vi "Query discriminator level.vi"(8 "error in (no error)":errorcluster, 10 "i (0)":T1, 11 "VISA resource name":refnum<visa-resource-name>) -> (0 "error out":errorcluster, 2 "output":dbl, 3 "VISA resource name out":refnum<visa-resource-name>)   [LabVIEW 2009, in "SR400.lvlib"]
doc: "DL i { ,v }\nThe DL command sets and reads the discriminator\nlevels. i = 0,1, or 2 designates discriminator A,B,\nor T and is required. If v is included, the selected\ndiscriminator level is set to v Volts where -0.3000\n<= V <= 0.3000. The resolution is 0.0002 V (0.2\nmV). If v is absent, the selected discriminator level\nis returned. If the discriminator mode is SCAN,\nthe DL command sets and reads the starting value\nof the level. Changing the level during a scan will\ncause the level to be set to the new value on the\nnext count period. Note that the scan is not reset.\nReading the level during a scan always returns the\nstarting value, not the current value."
uses:
  SR400.lvlib
  Typedefs.llb/Counter.ctl
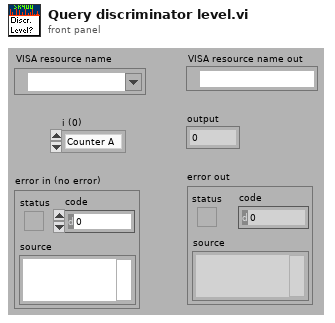
[diagram p1: front panel]
types:
  T1 = typedef "SR400.lvlib/Counter.ctl" = enum16{"Counter A", "Counter B", "Counter T"}
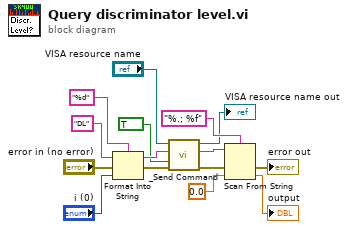
[diagram p0: block diagram]
diagram:
  n1 = Format Into String(format string="%d", initial string="DL" ("command"), error in="error in (no error)", "i (0)") -> (resulting string=w6:string, error out=w5:errorcluster)
  n2 = call "_Send Command.vi"("error in (no error)"=w5, "Query? (F)"=TRUE, "Command"=w6, "VISA resource name"="VISA resource name") -> ("error out"=w2:errorcluster, "Response"=w3:string, "VISA resource name out"=→"VISA resource name out":refnum<visa-resource-name>)  [unwired: 5 out]
  n3 = Scan From String(format string="%.; %f", input string=w3, error in=w2, default 1=0.0 ("default value 1")) -> (error out=→"error out":errorcluster, output 1=→"output":dbl)  [unwired: 1 in, 2 out]
